vi "New Set Camera Mode Message.vi"() -> (0 "Set Camera Mode Message":T1={"type"="camera_mode", "Vision Mode"={"message"="vision", "Active?"=TRUE}, "Intake Mode"={"message"="intake", "Active?"=FALSE}})   [LabVIEW 2016]
uses:
  Set Camera Mode Message.ctl
  Intake Mode.ctl
  Vision Mode.ctl
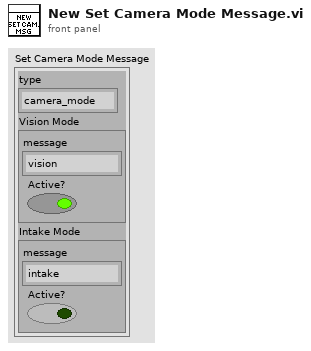
[diagram p1: front panel]
types:
  T1 = typedef "Set Camera Mode Message.ctl" = cluster{"type":string, "Vision Mode":cluster{"message":string, "Active?":bool}, "Intake Mode":cluster{"message":string, "Active?":bool}}
  T2 = typedef "Vision Mode.ctl" = cluster{"message":string, "Active?":bool}
  T3 = typedef "Intake Mode.ctl" = cluster{"message":string, "Active?":bool}
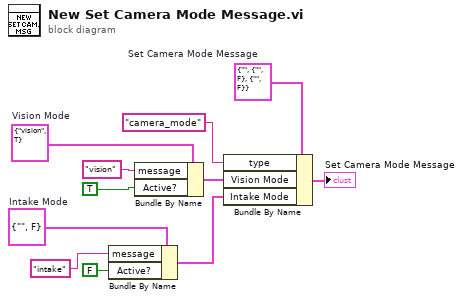
[diagram p0: block diagram]
diagram:
  w2 = T2 {"message"="vision", "Active?"=TRUE}  # Vision Mode
  w3 = T1 {"type"="", "Vision Mode"={"message"="", "Active?"=FALSE}, "Intake Mode"={"message"="", "Active?"=FALSE}}  # Set Camera Mode Message
  w7 = T3 {"message"="", "Active?"=FALSE}  # Intake Mode
  n1 = Bundle By Name(cluster=w7, "message"="intake" ("Message"), "Active?"=FALSE) -> (w4:T3)
  n2 = Bundle By Name(cluster=w2, "message"="vision" ("Message"), "Active?"=TRUE) -> (w8:T2)
  n3 = Bundle By Name(cluster=w3, "type"="camera_mode" ("Type"), "Vision Mode"=w8, "Intake Mode"=w4) -> (→"Set Camera Mode Message":T1)
